vi "Counter.vi"() -> ()   [LabVIEW 2010]
uses:
  libdaqVI.lvlib
panel:
  in  "退出程序":bool
  in  "选项卡控件":enum32{"CNT1", "CNT2"}(tab)
  out "占空比(%)":u32
  in  "mode":T1(ring) caption="测量模式"
  in  "cnt1_config":bool
  in  "cnt1_start":bool
  in  "cnt1_stop":bool
  in  "cnt1_clear":bool
  out "period":u32 caption="周期(ns)"
  out "计数值":u32
  out "pulse":u32 caption="脉冲宽度(ns)"
  in  "触发计数沿":T2(ring)
  out "占空比2(%)":u32 caption="占空比(%)"
  in  "cnt2_clear":bool
  out "period 2":u32 caption="周期(ns)"
  out "pulse 2":u32 caption="脉冲宽度(ns)"
  out "计数值":u32
  in  "cnt2_stop":bool
  in  "cnt2_start":bool
  in  "mode":T1(ring) caption="测量模式"
  in  "cnt2_config":bool
  in  "触发计数沿":T2(ring)
  out "状态":bool
  out "设备名称":string
  out "设备数量":u32
  # "范例说明：\n1、支持的采集卡：DAQ-USB3212、DAQ-USB3213、DAQ-USB3214\n2、CNT1和CNT2两个模块支持测量模式，包含计数测量 ，周期测量，PWM测量三种模式；CNT3和CNT4三种模块，支持发生器模式，包括PWM发生和脉冲发生两种模式；\n\n注意：\n1、无论测量模式和发生器模式，都会产生单片机的中断，因此测量的输入信号频率和产生的信号频率不建议超过100kHz；\n2、ADC模块的波形采样、DAC模块的波形输出工作过程也会产生单片机的中断，当单片机中断过于频繁会造成上位机下发的指令得不到响应，采集卡死机的假象，因此当与这些模块同时使用时，计数模块、ADC和DAC模块的工作频率需要进一步降低；\n3、采集卡包含ADC、DAC、CNT1、CNT2、CNT3、CNT4总共6个模块，建议同时使用的模块不要超过3个，具体以测试为准\n4、计数模块中周期和脉冲宽度的单位为纳秒(ns)"
  # "计数模块演示程序"
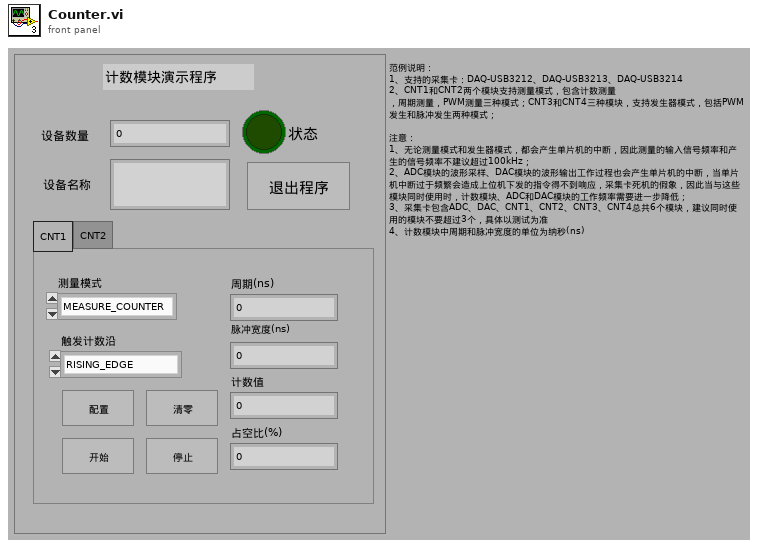
[diagram p1: front panel]
types:
  T1 = enum16{"MEASURE_COUNTER", "MEASURE_PERIOD", "MEASURE_PWM"}
  T2 = enum16{"RISING_EDGE", "FALLING_EDGE", "BOTH_EDGE"}
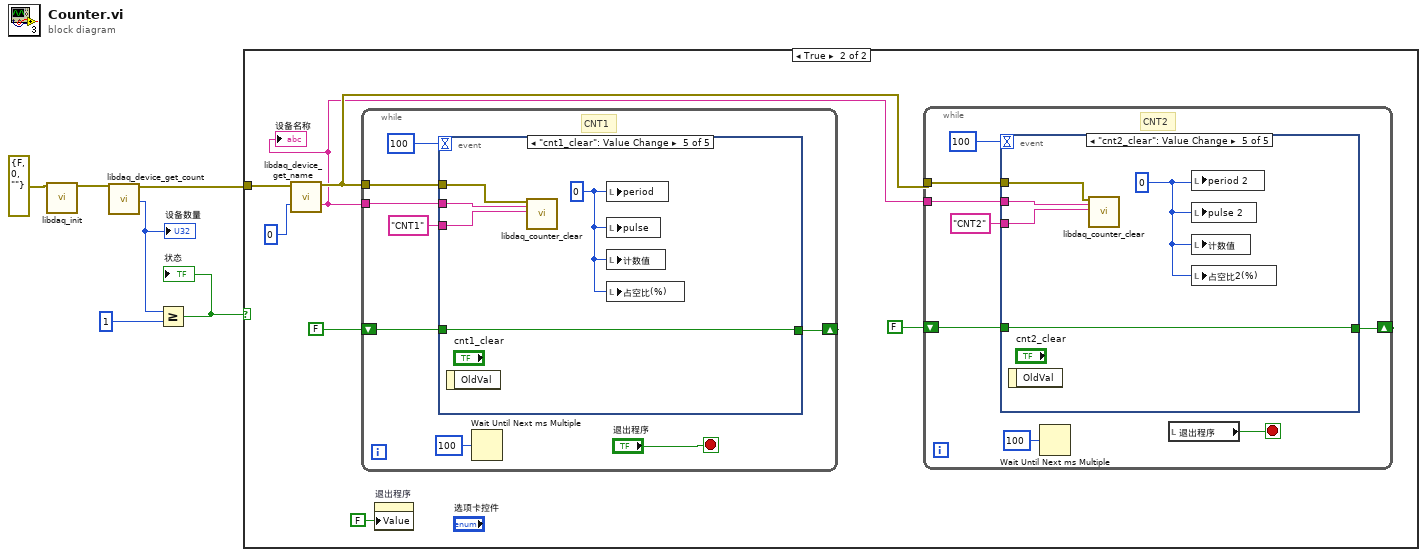
[diagram p0: block diagram]
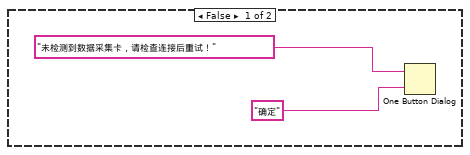
[diagram p2: hidden frame]
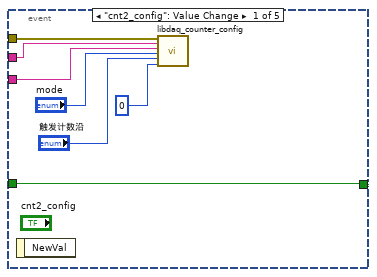
[diagram p3: hidden frame]
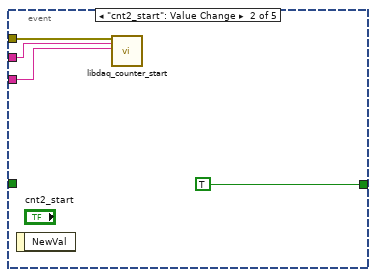
[diagram p4: hidden frame]
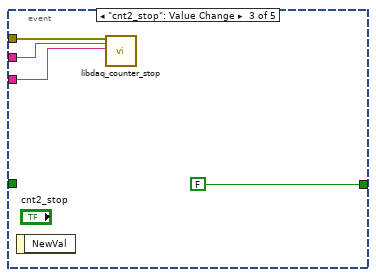
[diagram p5: hidden frame]
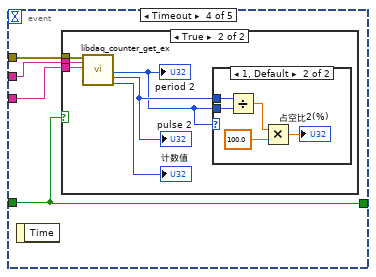
[diagram p6: hidden frame]
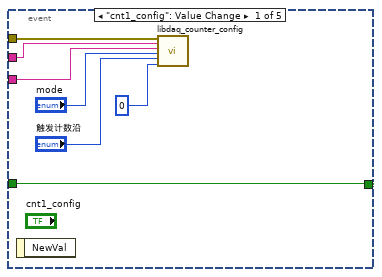
[diagram p9: hidden frame]
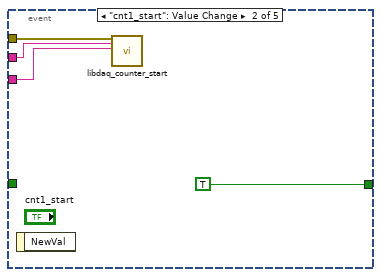
[diagram p10: hidden frame]
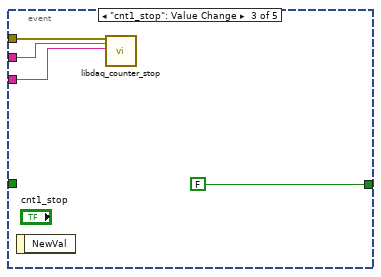
[diagram p11: hidden frame]
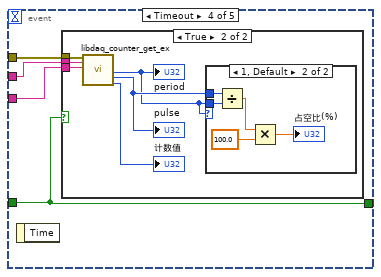
[diagram p12: hidden frame]
diagram:
  n1 = call "libdaq_init.vi"("error in (no error)"=errorcluster {"status"=FALSE, "code"=0, "source"=""}) -> ("error out"=w2:errorcluster)  [unwired: 18 in]
  n2 = call "libdaq_device_get_count.vi"("error in (no error)"=w2) -> ("error out"=w3:errorcluster, "device_count"=w1:i32)  [unwired: 17 in]
  "设备数量" <- w1
  n3 = Greater Or Equal?(x=w1, y=u32 1 ("name length")) -> (x >= y?=w5:bool)
  "状态" <- w5
  n4 = case shown="True" w5 {
    tunnel: w3 -> [_ w15]
    frame False {
      n5 = One Button Dialog(message="未检测到数据采集卡，请检查连接后重试！" ("消息"), button name ("OK")="确定" ("按钮名称（“确定”）")) -> ()  [unwired: 1 out]
    }
    frame True {
      n6 = call "libdaq_device_get_name.vi"("error in (no error)"=w15, "device_index"=u32 0 ("name length")) -> ("error out"=w11:errorcluster, "device_name"=w10:string)  [unwired: 16 in]
      "设备名称" <- w10
      n7 = while {
        tunnel: w11 -> [w65]
        tunnel: w10 -> [w64]
        shift-right: [w61] -> _
        shift-left: FALSE -> [w62]
        stop <- "退出程序" stop-if-true
        # "CNT1"
        n8 = event shown="[4] \"cnt1_clear\": Value Change" {
          selector: _ -> [_ _ _ _ _]
          dyn-events: _ -> [_ _ _ _ _]
          timeout: 100 -> [_ _ _ _ _]
          tunnel: w65 -> [w73 w77 w81 w85 w101]
          tunnel: w64 -> [w72 w76 w80 w84 w100]
          tunnel: "CNT1" ("module_name") -> [w69 w75 w79 w83 w99]
          tunnel: w62 -> [w68 _ _ w82 w98]
          tunnel: [w68 TRUE FALSE w82 w98] -> w61
          event "cnt1_config": Value Change {
            n9 = event-data() -> ()  [unwired: 1 in, 1 out]
            n10 = call "libdaq_counter_config.vi"("error in (no error)"=w73, "device_name"=w72, "module_name"=w69, "mode"="mode", "edge"="触发计数沿", "period"=0) -> ()  [unwired: 11 in, 3 out]
          }
          event "cnt1_start": Value Change {
            n11 = event-data() -> ()  [unwired: 1 in, 1 out]
            n12 = call "libdaq_counter_start.vi"("error in (no error)"=w77, "device_name"=w76, "module_name"=w75) -> ()  [unwired: 14 in, 3 out]
          }
          event "cnt1_stop": Value Change {
            n13 = event-data() -> ()  [unwired: 1 in, 1 out]
            n14 = call "libdaq_counter_stop.vi"("error in (no error)"=w81, "device_name"=w80, "module_name"=w79) -> ()  [unwired: 14 in, 3 out]
          }
          event Timeout {
            n15 = event-data() -> ()  [unwired: 1 in, 1 out]
            n16 = case shown="True" w82 {
              tunnel: w85 -> [_ w91]
              tunnel: w84 -> [_ w90]
              tunnel: w83 -> [_ w89]
              frame False {
              }
              frame True {
                n17 = call "libdaq_counter_get_ex.vi"("error in (no error)"=w91, "device_name"=w90, "module_name"=w89) -> ("period"=w86:u32, "pulse"=w87:u32, "count"=→"计数值":u32)  [unwired: 11 in, 3 out]
                "period" <- w86
                "pulse" <- w87
                n18 = case shown="1, Default" w86 {
                  tunnel: w87 -> [_ w96]
                  tunnel: w86 -> [_ w95]
                  frame 0 {
                  }
                  frame 1, Default {
                    n19 = Divide(x=w96, y=w95) -> (x/y=w94:dbl)
                    n20 = Multiply(x=w94, y=100.0) -> (x*y=→"占空比(%)":dbl)
                  }
                }
              }
            }
          }
          event "cnt1_clear": Value Change {
            w97 = u32 0 ("period")
            n21 = event-data() -> ()  [unwired: 1 in, 1 out]
            n22 = call "libdaq_counter_clear.vi"("error in (no error)"=w101, "device_name"=w100, "module_name"=w99) -> ()  [unwired: 14 in, 3 out]
            n23 = local write "period"(w97) -> ()
            n24 = local write "pulse"(w97) -> ()
            n25 = local write "计数值"(w97) -> ()
            n26 = local write "占空比(%)"(w97) -> ()
          }
        }
        n27 = Wait Until Next ms Multiple(millisecond multiple=u32 100 ("毫秒倍数")) -> ()  [unwired: 1 out]
      }
      n28 = property on="退出程序" class="Bool (strict)"("Value"=FALSE ("退出程序")) -> ()  [unwired: 2 in, 2 out]
      n29 = while {
        tunnel: w11 -> [w22]
        tunnel: w10 -> [w21]
        shift-right: [w18] -> _
        shift-left: FALSE -> [w19]
        stop <- w17 stop-if-true
        # "CNT2"
        n30 = event shown="[4] \"cnt2_clear\": Value Change" {
          selector: _ -> [_ _ _ _ _]
          dyn-events: _ -> [_ _ _ _ _]
          timeout: 100 -> [_ _ _ _ _]
          tunnel: w22 -> [w30 w34 w38 w42 w58]
          tunnel: w21 -> [w29 w33 w37 w41 w57]
          tunnel: "CNT2" ("module_name") -> [w26 w32 w36 w40 w56]
          tunnel: w19 -> [w25 _ _ w39 w55]
          tunnel: [w25 TRUE FALSE w39 w55] -> w18
          event "cnt2_config": Value Change {
            n31 = event-data() -> ()  [unwired: 1 in, 1 out]
            n32 = call "libdaq_counter_config.vi"("error in (no error)"=w30, "device_name"=w29, "module_name"=w26, "mode"="mode", "edge"="触发计数沿", "period"=0) -> ()  [unwired: 11 in, 3 out]
          }
          event "cnt2_start": Value Change {
            n33 = event-data() -> ()  [unwired: 1 in, 1 out]
            n34 = call "libdaq_counter_start.vi"("error in (no error)"=w34, "device_name"=w33, "module_name"=w32) -> ()  [unwired: 14 in, 3 out]
          }
          event "cnt2_stop": Value Change {
            n35 = event-data() -> ()  [unwired: 1 in, 1 out]
            n36 = call "libdaq_counter_stop.vi"("error in (no error)"=w38, "device_name"=w37, "module_name"=w36) -> ()  [unwired: 14 in, 3 out]
          }
          event Timeout {
            n37 = event-data() -> ()  [unwired: 1 in, 1 out]
            n38 = case shown="True" w39 {
              tunnel: w42 -> [_ w48]
              tunnel: w41 -> [_ w47]
              tunnel: w40 -> [_ w46]
              frame False {
              }
              frame True {
                n39 = call "libdaq_counter_get_ex.vi"("error in (no error)"=w48, "device_name"=w47, "module_name"=w46) -> ("period"=w43:u32, "pulse"=w44:u32, "count"=→"计数值":u32)  [unwired: 11 in, 3 out]
                "period 2" <- w43
                "pulse 2" <- w44
                n40 = case shown="1, Default" w43 {
                  tunnel: w44 -> [_ w53]
                  tunnel: w43 -> [_ w52]
                  frame 0 {
                  }
                  frame 1, Default {
                    n41 = Divide(x=w53, y=w52) -> (x/y=w49:dbl)
                    n42 = Multiply(x=w49, y=100.0) -> (x*y=→"占空比2(%)":dbl)
                  }
                }
              }
            }
          }
          event "cnt2_clear": Value Change {
            w54 = u32 0 ("period")
            n43 = event-data() -> ()  [unwired: 1 in, 1 out]
            n44 = call "libdaq_counter_clear.vi"("error in (no error)"=w58, "device_name"=w57, "module_name"=w56) -> ()  [unwired: 14 in, 3 out]
            n45 = local write "period 2"(w54) -> ()
            n46 = local write "pulse 2"(w54) -> ()
            n47 = local write "计数值"(w54) -> ()
            n48 = local write "占空比2(%)"(w54) -> ()
          }
        }
        n49 = Wait Until Next ms Multiple(millisecond multiple=u32 100 ("毫秒倍数")) -> ()  [unwired: 1 out]
        n50 = local read "退出程序"() -> (w17:bool)
      }
    }
  }
